vi "SequenceIndex.vi"(10 "Steps":u32=1, 11 "SequenceIndexName":string) -> (3 "SequenceIndex":refnum<class "SequenceIndex.lvclass">)   [LabVIEW 2013, in "VariableManagerAPI.lvlib"]
doc: "Return Sequence index definition object.\nThe object contains given values (optional).\nData can be accessed through property node.\n\n<B>SequenceIndexName</B>: the name of the sequence index\n<B>Steps</B>: the number of steps of the sequence index"
uses:
  VariableManagerAPI.lvlib
  SequenceIndex/SequenceIndex.lvclass
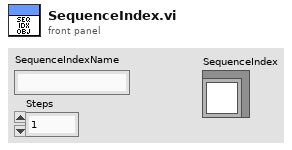
[diagram p1: front panel]
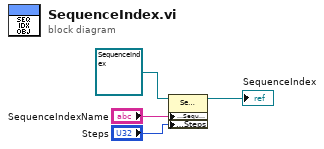
[diagram p0: block diagram]
diagram:
  n1 = property class="SequenceIndex.lvclass"(reference=refnum<class "SequenceIndex.lvclass"> refnum ("SequenceIndex.lvclass"), "Accessors:SequenceIndexName"="SequenceIndexName", "Accessors:Steps"="Steps") -> (reference out=→"SequenceIndex":refnum<class "SequenceIndex.lvclass">)  [unwired: 1 in, 1 out]
